vi "Curtin_CleanConfigString.vi"(11 "String in":string) -> (3 "String out":string)   [LabVIEW 2022 SP3]
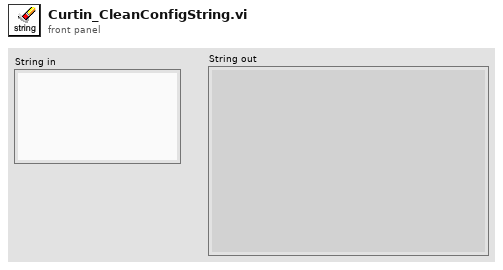
[diagram p1: front panel]
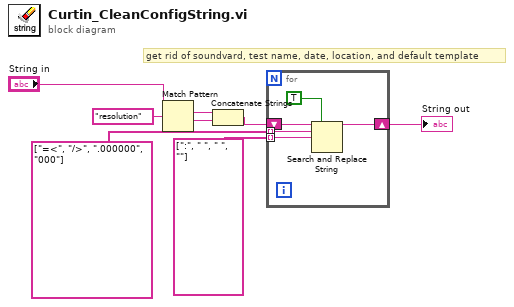
[diagram p0: block diagram]
diagram:
  # "get rid of soundvard, test name, date, location, and default template"
  n1 = Match Pattern(string="String in", regular expression="resolution") -> (match substring=w3:string, after substring=w4:string)  [unwired: 1 in, 2 out]
  n2 = Concatenate Strings(w3, w4) -> (w5:string)
  n3 = for {
    shift-right: [w12] -> w6
    shift-left: w5 -> [w13]
    tunnel: string[] ["=<", "/>", ".000000", "000"] -> [w10] mode=indexing
    tunnel: string[] [":", " ", " ", ""] -> [w9] mode=indexing
    n4 = Search and Replace String(replace all?=TRUE ("replace all? (F)"), input string=w13, search string=w10, replace string=w9) -> (result string=w12:string)  [unwired: 4 in, 3 out]
  }
  "String out" <- w6
